vi "Element Events.vi"(8 "error in (no error)":errorcluster, 11 "SystemConfigStatusIndicator in":refnum<class "SystemConfigStatusIndicator.lvclass">) -> (0 "error out":errorcluster, 2 "Element Events":refnum<class "Control Event Registrations.lvclass">, 3 "SystemConfigStatusIndicator out":refnum<class "SystemConfigStatusIndicator.lvclass">)   [LabVIEW 2020, in "VolatusGUIElements.lvlib" / "SystemConfigStatusIndicator.lvclass"]
uses:
  SystemConfigStatusIndicator.lvclass
  VolatusGUI/Control Event Registrations/Control Event Registrations.lvclass
  SystemConfigStatusIndicator.lvclass/SystemConfigStatusIndicator.ctl
  VolatusGUI/GUI Element/GUI Element.lvclass
  C:/dev/lv20CE/relink/lv-volatus/VolatusGUI/GUI Element/GUI Element.lvclass
  C:/dev/lv20CE/relink/lv-volatus/VolatusGUIElements/SystemConfigStatusIndicator/SystemConfigStatusIndicator.lvclass
  C:/dev/lv20CE/relink/lv-volatus/VolatusGUI/OnValueChangeHandler/OnValueChangeHandler.lvclass
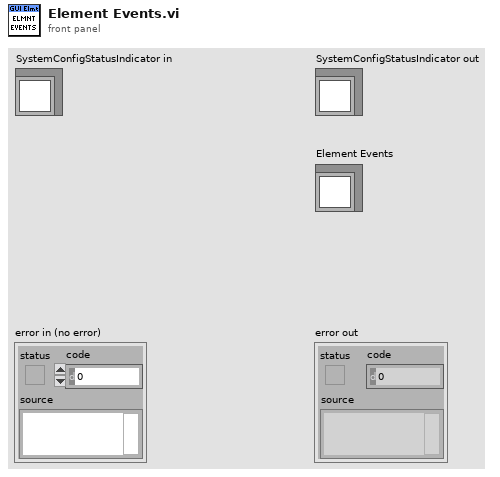
[diagram p1: front panel]
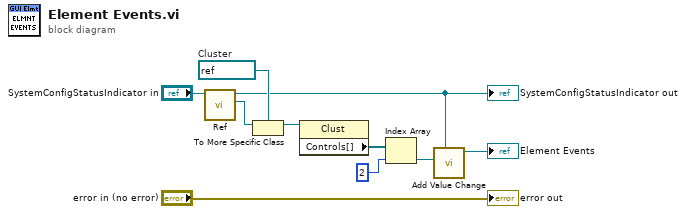
[diagram p0: block diagram]
diagram:
  w7 = refnum<vi> refnum  # Cluster
  n1 = call "Ref.vi"("GUI Element in"="SystemConfigStatusIndicator in") -> ("Ref"=w8:refnum<vi>, "GUI Element out"=w2:refnum<class "SystemConfigStatusIndicator.lvclass">)  [unwired: 9 in]
  "SystemConfigStatusIndicator out" <- w2
  n2 = To More Specific Class(target class=w7, reference=w8) -> (specific class reference=w6:refnum<vi>)  [unwired: 1 in, 1 out]
  n3 = property class="Clust"(reference=w6) -> ("Controls[]"=w5:refnum<vi>[])  [unwired: 1 in, 2 out]
  n4 = Index Array(array=w5, index=2) -> (element=w3:refnum<vi>)
  n5 = call "Add Value Change.vi"("Control"=w2, "CtlRef"=w3) -> ("Control Event Registrations out"=→"Element Events":refnum<class "Control Event Registrations.lvclass">)  [unwired: 8 in, 1 out]
  "error out" <- "error in (no error)"
